vi "Disconnect CAN Adapter.vi"(8 "error in":errorcluster, 11 "CANopen Master in":refnum<class "CANopen Master.lvclass">) -> (0 "error out":errorcluster, 3 "CANopen Master out":refnum<class "CANopen Master.lvclass">)   [LabVIEW 2024, in "CANopen Master.lvlib" / "CANopen Master.lvclass"]
uses:
  CANopen Master.lvclass
  HAL/Source/Interfaces/IClose/IClose.lvclass
  CANopen Master.lvclass/CANopen Master.ctl
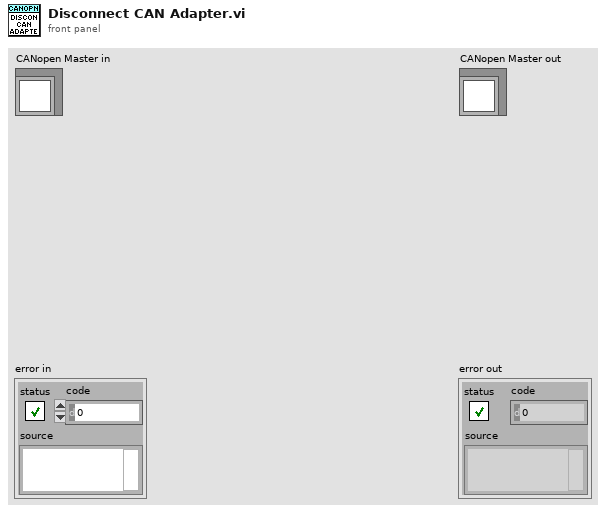
[diagram p1: front panel]
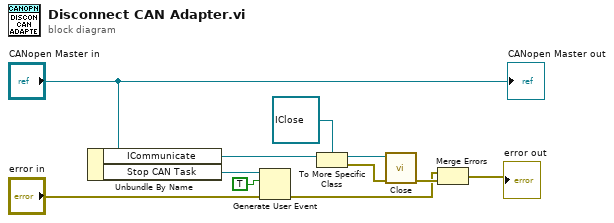
[diagram p0: block diagram]
diagram:
  n1 = Unbundle By Name("CANopen Master in") -> ("ICommunicate"=w8:refnum<class "ICommunicate.lvclass">, "Stop CAN Task"=w9:refnum<user-event>)
  n2 = Generate User Event(user event=w9, event data cluster=TRUE ("event data"), error in="error in") -> (error out=w1:errorcluster)  [unwired: 1 in, 1 out]
  n3 = To More Specific Class(target class=refnum<class "IClose.lvclass"> refnum ("IClose.lvclass"), reference=w8) -> (specific class reference=w6:refnum<class "IClose.lvclass">, error out=w5:errorcluster)  [unwired: 1 in]
  n4 = call-dynamic "Close.vi"("error in"=w5, "IClose in"=w6) -> ("error out"=w4:errorcluster)  [unwired: 8 in, 1 out]
  n5 = Merge Errors(w1, w4) -> (→"error out":errorcluster)
  "CANopen Master out" <- "CANopen Master in"
